vi "test_data.vi"() -> ()   [LabVIEW 2021]
uses:
  Parent/Parent.lvclass
  Child/Child.lvclass
panel:
  out "message 3":string
  out "message 2":string
  out "message 1":string
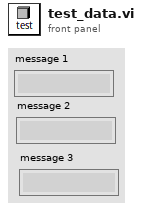
[diagram p1: front panel]
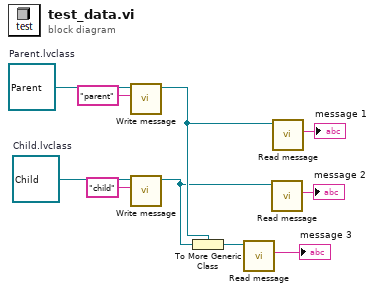
[diagram p0: block diagram]
diagram:
  w8 = refnum<class "Child.lvclass"> refnum  # Child.lvclass
  w10 = refnum<class "Parent.lvclass"> refnum  # Parent.lvclass
  n1 = call-dynamic "Write message.vi"("message"="parent", "Parent in"=w10) -> ("Parent out"=w6:refnum<class "Parent.lvclass">)  [unwired: 8 in, 1 out]
  n2 = call-dynamic "Write message.vi"("message"="child", "Child in"=w8) -> ("Child out"=w4:refnum<class "Child.lvclass">)  [unwired: 8 in, 1 out]
  n3 = To More Generic Class(target class=w6, reference=w4) -> (generic class reference=w2:refnum<class "Parent.lvclass">)
  n4 = call-dynamic "Read message.vi"("Parent in"=w2) -> ("message"=→"message 3":string)  [unwired: 8 in, 2 out]
  n5 = call-dynamic "Read message.vi"("Child in"=w4) -> ("message"=→"message 2":string)  [unwired: 8 in, 2 out]
  n6 = call-dynamic "Read message.vi"("Parent in"=w6) -> ("message"=→"message 1":string)  [unwired: 8 in, 2 out]
